vi "ShipShootTiming.vi"(7 "Selector":T1, 11 "ShootEnergy":dbl=2000.0 format="%#_13g") -> (2 "Time":u32, 3 "Ready2Shoot":bool)   [LabVIEW 2022 SP3]
uses:
  ShipShootEnum.ctl
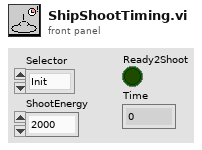
[diagram p1: front panel]
types:
  T1 = typedef "ShipShootEnum.ctl" = enum16{"Init", "Read", "Reset"}
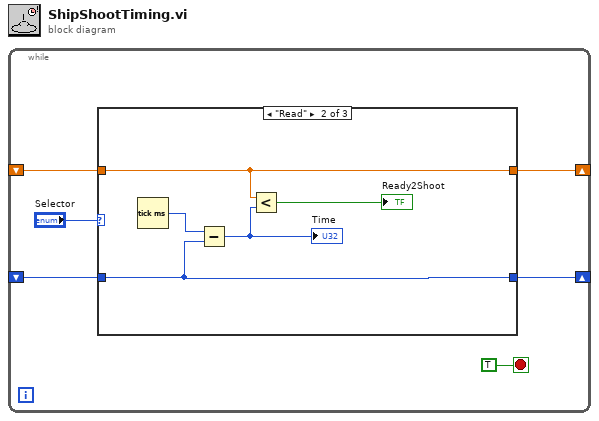
[diagram p0: block diagram]
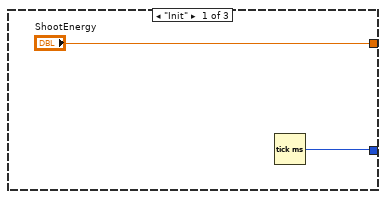
[diagram p2: hidden frame]
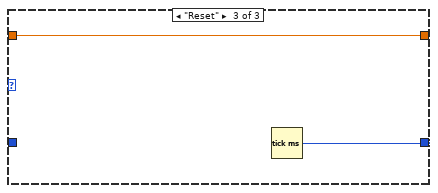
[diagram p3: hidden frame]
diagram:
  n1 = while {
    shift-right: [w4] -> _
    shift-left: _ -> [w3]
    shift-right: [w2] -> _
    shift-left: _ -> [w1]
    stop <- TRUE stop-if-true
    n2 = case shown="\"Read\"" "Selector" {
      tunnel: ["ShootEnergy" w12 w14] -> w4
      tunnel: w3 -> [_ w12 w14]
      tunnel: [w7 w9 w15] -> w2
      tunnel: w1 -> [_ w9 _]
      frame "Init" {
        n3 = Tick Count (ms)() -> (millisecond timer value=w7:u32)
      }
      frame "Read" {
        n4 = Tick Count (ms)() -> (millisecond timer value=w13:u32)
        n5 = Subtract(x=w13, y=w9) -> (x-y=w11:u32)
        "Time" <- w11
        n6 = Less?(x=w12, y=w11) -> (x < y?=→"Ready2Shoot":bool)
      }
      frame "Reset" {
        n7 = Tick Count (ms)() -> (millisecond timer value=w15:u32)
      }
    }
  }
